vi "CalcBouncerGate.lestates.vi"(9 "Bouncer Settings":T1 {"LE12C Voltage" format="%_4f"; "LE13C Voltage" format="%_4f"}, 10 "SampClk.Rate":dbl) -> (1 "Bouncer Waveform":waveform(dbl), 2 "High time":dbl, 3 "low time":dbl)   [LabVIEW 2011]
uses:
  BouncerParameters.ctl
panel:
  # "ms"
  # "us"
  # "kV"
  # "ms"
  # "us"
  # "kV"
  # "ms"
  # "us"
  # "kV"
  # "ms"
  # "us"
  # "kV"
  # "ms"
  # "us"
  # "kV"
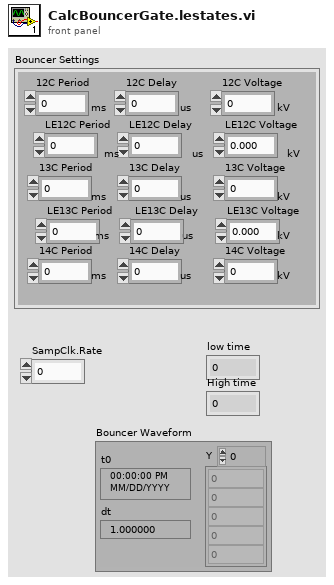
[diagram p1: front panel]
types:
  T1 = typedef "BouncerParameters.ctl" = cluster{"12C Period":dbl, "12C Delay":dbl, "12C Voltage":dbl, "13C Period":dbl, "13C Delay":dbl, "13C Voltage":dbl, "14C Period":dbl, "14C Delay":dbl, "14C Voltage":dbl, "LE13C Period":dbl, "LE13C Delay":dbl, "LE13C Voltage":dbl, "LE12C Period":dbl, "LE12C Delay":dbl, "LE12C Voltage":dbl}
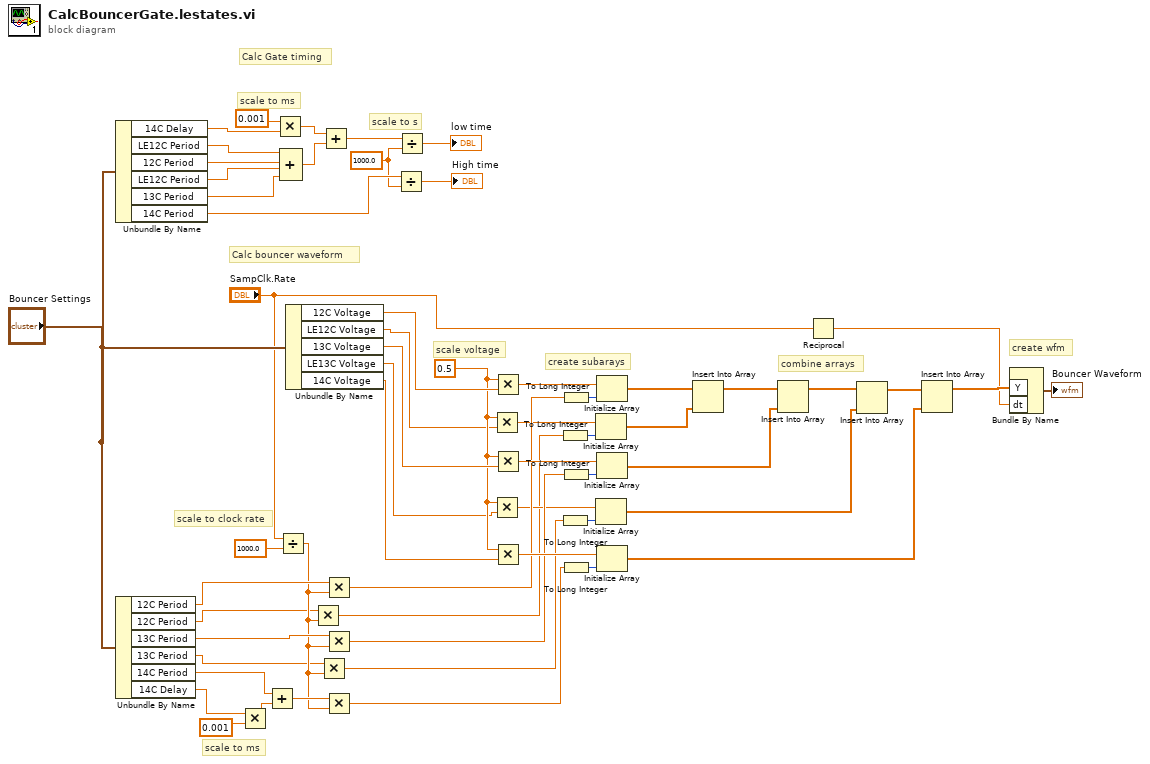
[diagram p0: block diagram]
diagram:
  w30 = 1000.0 ("y")
  w11 = 0.5 ("y")
  # "Calc bouncer waveform"
  # "Calc Gate timing"
  # "create wfm"
  # "combine arrays"
  # "create subarays"
  # "scale voltage"
  # "scale to clock rate"
  # "scale to ms"
  # "scale to s"
  # "scale to ms"
  n1 = Unbundle By Name("Bouncer Settings") -> ("14C Delay"=w28:dbl, "LE12C Period"=w33:dbl, "12C Period"=w21:dbl, "LE12C Period"=w20:dbl, "13C Period"=w19:dbl, "14C Period"=w34:dbl)
  n2 = Unbundle By Name("Bouncer Settings") -> ("12C Period"=w47:dbl, "12C Period"=w16:dbl, "13C Period"=w46:dbl, "13C Period"=w17:dbl, "14C Period"=w38:dbl, "14C Delay"=w35:dbl)
  n3 = Multiply(x=w35, y=0.001) -> (x*y=w36:dbl)
  n4 = Add(x=w38, y=w36) -> (x+y=w58:dbl)
  n5 = Multiply(x=0.001 ("y"), y=w28) -> (x*y=w32:dbl)
  n6 = Divide(x="SampClk.Rate", y=1000.0) -> (x/y=w18:dbl)
  n7 = Compound Arithmetic op=ADD(w33, w21, w20, w19) -> (w31:dbl)
  n8 = Unbundle By Name("Bouncer Settings") -> ("12C Voltage"=w45:dbl, "LE12C Voltage"=w10:dbl, "13C Voltage"=w44:dbl, "LE13C Voltage"=w9:dbl, "14C Voltage"=w43:dbl)
  n9 = Multiply(x=w16, y=w18) -> (x*y=w7:dbl)
  n10 = Multiply(x=w17, y=w18) -> (x*y=w8:dbl)
  n11 = Add(x=w32, y=w31) -> (x+y=w29:dbl)
  n12 = Multiply(x=w47, y=w18) -> (x*y=w51:dbl)
  n13 = Multiply(x=w46, y=w18) -> (x*y=w50:dbl)
  n14 = Multiply(x=w58, y=w18) -> (x*y=w49:dbl)
  n15 = Divide(x=w34, y=w30) -> (x/y=→"High time":dbl)
  n16 = Divide(x=w29, y=w30) -> (x/y=→"low time":dbl)
  n17 = Multiply(x=w11, y=w10) -> (x*y=w15:dbl)
  n18 = Multiply(x=w11, y=w9) -> (x*y=w13:dbl)
  n19 = Multiply(x=w11, y=w45) -> (x*y=w56:dbl)
  n20 = Multiply(x=w11, y=w44) -> (x*y=w55:dbl)
  n21 = Multiply(x=w11, y=w43) -> (x*y=w57:dbl)
  n22 = To Long Integer(number=w7) -> (32bit integer=w14:i32)
  n23 = To Long Integer(number=w8) -> (32bit integer=w12:i32)
  n24 = To Long Integer(number=w51) -> (32bit integer=w40:i32)
  n25 = To Long Integer(number=w50) -> (32bit integer=w41:i32)
  n26 = To Long Integer(number=w49) -> (32bit integer=w42:i32)
  n27 = Initialize Array(w15, w14) -> (w5:dbl[])
  n28 = Initialize Array(w13, w12) -> (w4:dbl[])
  n29 = Initialize Array(w56, w40) -> (w6:dbl[])
  n30 = Initialize Array(w55, w41) -> (w54:dbl[])
  n31 = Initialize Array(w57, w42) -> (w53:dbl[])
  n32 = Insert Into Array(array=w6, new element=w5) -> (w3:dbl[])  [unwired: 1 in]
  n33 = Insert Into Array(array=w3, new element=w54) -> (w2:dbl[])  [unwired: 1 in]
  n34 = Reciprocal(x="SampClk.Rate") -> (1/x=w48:dbl)
  n35 = Insert Into Array(array=w2, new element=w4) -> (w1:dbl[])  [unwired: 1 in]
  n36 = Insert Into Array(array=w1, new element=w53) -> (w52:dbl[])  [unwired: 1 in]
  n37 = Bundle By Name("Y"=w52, "dt"=w48) -> (→"Bouncer Waveform":waveform(dbl))  [unwired: 1 out]
